vi "SwerveDrive2.vi"(8 "error in":errorcluster) -> (0 "error out":errorcluster)   [LabVIEW 2016]
uses:
  Refname/Motors.ctl
  Main/Robot Global Data.vi
  Refname/Refname to String (Motors).vi
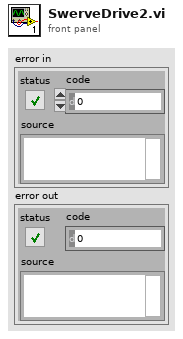
[diagram p1: front panel]
types:
  T1 = typedef "Motors.ctl" = enum16{"Wheel 1", "Swerve 1", "Wheel 2", "Swerve 2", "Wheel 3", "Swerve 3", "Wheel 4", "Swerve 4"}
  T2 = typedef "WPI_MotorControlDeviceRef.ctl" = cluster{"DeviceStatus":errorcluster, "Type":T3, "PWM":cluster{"PWM Channel":T4, "DeadBand":T5}, "CAN":cluster{"Device Number":u8, "SetOutput VI Ref":variant, "GetOutput VI Ref":variant, "Enable VI Ref":variant, "Disable VI Ref":variant, "Data":variant}, "Invert":bool}
  T3 = typedef "WPI_MotorControlType.ctl" = enum16{"PWM", "CAN"}
  T4 = typedef "FPGA_DIOPWMChannel.ctl" = enum8{"PWM 0", "PWM 1", "PWM 2", "PWM 3", "PWM 4", "PWM 5", "PWM 6", "PWM 7", "PWM 8", "PWM 9", "PWM MXP 0", "PWM MXP 1", "PWM MXP 2", "PWM MXP 3", "PWM MXP 4", "PWM MXP 5", "PWM MXP 6", "PWM MXP 7", "PWM MXP 8", "PWM MXP 9", "Invalid"}
  T5 = typedef "WPI_PWMDeadband.ctl" = cluster{"Name":string, "maxPositivePwm":i32, "minPositivePwm":i32, "centerPwm":i32, "maxNegativePwm":i32, "minNegativePwm":i32, "angularRange":u16}
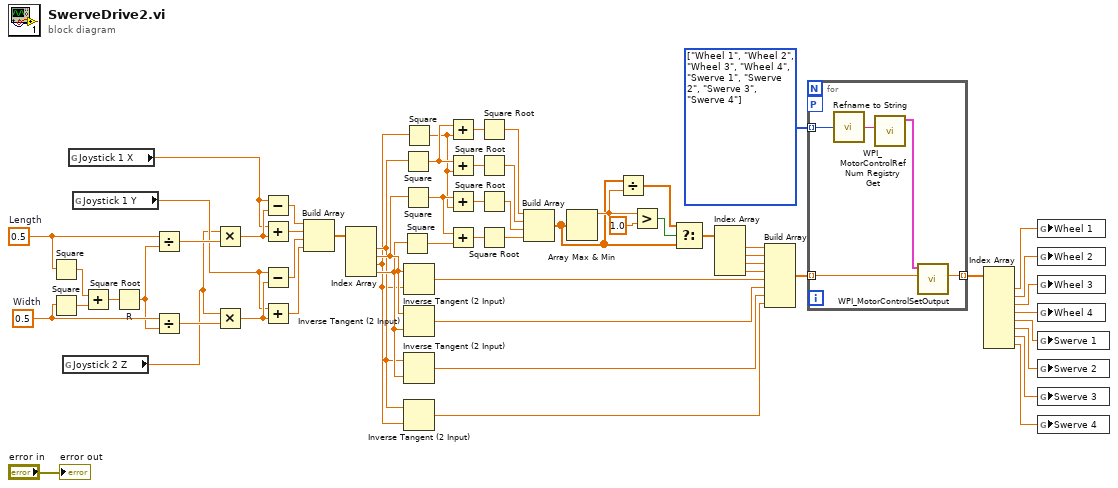
[diagram p0: block diagram]
diagram:
  w24 = T1[] [enum."Wheel 1", enum."Wheel 2", enum."Wheel 3", enum."Wheel 4", enum."Swerve 1", enum."Swerve 2", enum."Swerve 3", enum."Swerve 4"] items=["Wheel 1", "Swerve 1", "Wheel 2", "Swerve 2", "Wheel 3", "Swerve 3", "Wheel 4", "Swerve 4"]
  w52 = 0.5  # Width
  w56 = 0.5  # Length
  n1 = Square(x=w56) -> (x^2=w60:dbl)
  n2 = Square(x=w52) -> (x^2=w59:dbl)
  n3 = global read "Robot Global Data.vi" "Joystick 2 Z"() -> (w1:dbl)
  n4 = global read "Robot Global Data.vi" "Joystick 1 X"() -> (w3:dbl)
  n5 = global read "Robot Global Data.vi" "Joystick 1 Y"() -> (w2:dbl)
  n6 = Add(x=w60, y=w59) -> (x+y=w58:dbl)
  n7 = Square Root "R"(x=w58) -> (sqrt(x)=w51:dbl)
  n8 = Divide(x=w56, y=w51) -> (x/y=w57:dbl)
  n9 = Divide(x=w52, y=w51) -> (x/y=w50:dbl)
  n10 = Multiply(x=w1, y=w57) -> (x*y=w54:dbl)
  n11 = Multiply(x=w1, y=w50) -> (x*y=w48:dbl)
  n12 = Subtract(x=w3, y=w54) -> (x-y=w55:dbl)
  n13 = Add(x=w3, y=w54) -> (x+y=w53:dbl)
  n14 = Subtract(x=w2, y=w48) -> (x-y=w49:dbl)
  n15 = Add(x=w2, y=w48) -> (x+y=w47:dbl)
  n16 = Build Array(w55, w53, w49, w47) -> (w46:dbl[])
  n17 = Index Array(array=w46) -> (element #1=w26:dbl, element #2=w28:dbl, element #3=w25:dbl, element #4=w27:dbl)  [unwired: 4 in]
  n18 = Square(x=w27) -> (x^2=w43:dbl)
  n19 = Square(x=w26) -> (x^2=w39:dbl)
  n20 = Square(x=w28) -> (x^2=w44:dbl)
  n21 = Square(x=w25) -> (x^2=w38:dbl)
  n22 = Inverse Tangent (2 Input)(1:w25, 2:w28) -> (0:w18:dbl)
  n23 = Inverse Tangent (2 Input)(1:w27, 2:w28) -> (0:w17:dbl)
  n24 = Inverse Tangent (2 Input)(1:w27, 2:w26) -> (0:w16:dbl)
  n25 = Inverse Tangent (2 Input)(1:w25, 2:w26) -> (0:w15:dbl)
  n26 = Add(x=w39, y=w38) -> (x+y=w41:dbl)
  n27 = Add(x=w39, y=w38) -> (x+y=w40:dbl)
  n28 = Add(x=w44, y=w38) -> (x+y=w45:dbl)
  n29 = Add(x=w44, y=w43) -> (x+y=w42:dbl)
  n30 = Square Root(x=w41) -> (sqrt(x)=w37:dbl)
  n31 = Square Root(x=w40) -> (sqrt(x)=w36:dbl)
  n32 = Square Root(x=w45) -> (sqrt(x)=w35:dbl)
  n33 = Square Root(x=w42) -> (sqrt(x)=w34:dbl)
  n34 = Build Array(w37, w36, w35, w34) -> (w29:dbl[])
  n35 = Array Max & Min(array=w29) -> (max value=w31:dbl)  [unwired: 3 out]
  n36 = Divide(x=w29, y=w31) -> (x/y=w30:dbl[])
  n37 = Greater?(x=w31, y=1.0) -> (0:w32:bool)
  n38 = Select(t=w30, s=w32, f=w29) -> (s? t:f=w23:dbl[])
  n39 = Index Array(array=w23) -> (element #1=w22:dbl, element #2=w21:dbl, element #3=w20:dbl, element #4=w19:dbl)  [unwired: 4 in]
  n40 = Build Array(w22, w21, w20, w19, w18, w17, w16, w15) -> (w14:dbl[])
  n41 = for {
    workers-P: _ -> [_]
    tunnel: w24 -> [w65] mode=indexing
    tunnel: w14 -> [w62] mode=indexing
    tunnel: [w61] -> w12 mode=indexing
    n42 = call-poly "Refname to String.vi"("Enum"=w65) -> ("String"=w64:string)
    n43 = call <vilib>:"WPI_MotorControlRefNum Registry Get.vi"("refnum name"=w64) -> ("MotorControlDevRef"=w63:T2)  [unwired: 9 in, 1 out]
    n44 = call <vilib>:"WPI_MotorControlSetOutput.vi"("Output"=w62, "MotorControlDevRef"=w63) -> ("Motor Output"=w61:dbl)  [unwired: 7 in, 2 out]
  }
  n45 = Index Array(array=w12) -> (element #1=w11:dbl, element #2=w10:dbl, element #3=w9:dbl, element #4=w8:dbl, element #5=w7:dbl, element #6=w6:dbl, element #7=w5:dbl, element #8=w4:dbl)  [unwired: 8 in]
  n46 = global write "Robot Global Data.vi" "Wheel 1"(w11) -> ()
  n47 = global write "Robot Global Data.vi" "Wheel 2"(w10) -> ()
  n48 = global write "Robot Global Data.vi" "Wheel 3"(w9) -> ()
  n49 = global write "Robot Global Data.vi" "Wheel 4"(w8) -> ()
  n50 = global write "Robot Global Data.vi" "Swerve 1"(w7) -> ()
  n51 = global write "Robot Global Data.vi" "Swerve 2"(w6) -> ()
  n52 = global write "Robot Global Data.vi" "Swerve 3"(w5) -> ()
  n53 = global write "Robot Global Data.vi" "Swerve 4"(w4) -> ()
  "error out" <- "error in"
